vi "Update FormulaG Project.vi"() -> ()   [LabVIEW 2020]
uses:
  dev/Version.ctl
  dev/Updater State.ctl
  c5f3ca88-f85c-4b21-a54c-2e2b82621a56.vi
  fab92dee-f5cc-474f-8dc6-a01214f8643b.vi
  <vilib>/Comparison/Equal/Equal Functor/Equal Functor.lvclass
panel:
  out "Web Folder":path
  out "Project":refnum<vi>
  out "Template Vers Str":string
  out "Project Vers Str":string
  out "Template Version":T1
  out "Project Version":T1
  out "Common Folder":path
  out "Progress":u16(slide) scale=0.0..100.0
  out "Status":string
  out "Players":path[](array[path])
  out "Template":path
  out "Engine Folder":path
  out "Project Path":path
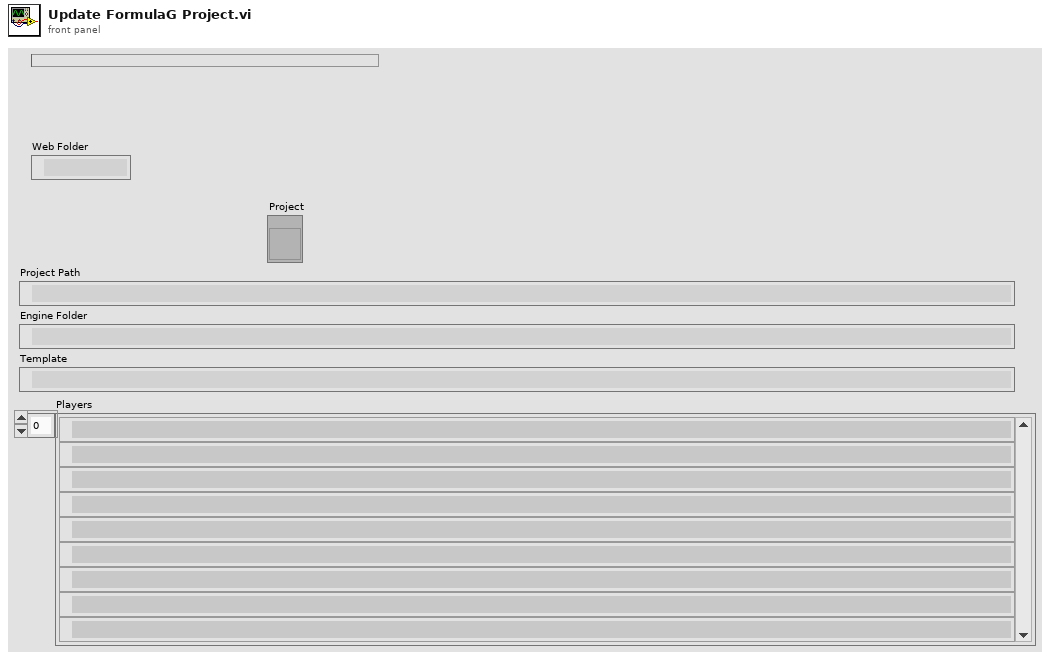
[diagram p1: front panel]
types:
  T1 = typedef "Version.ctl" = cluster{"Major":u16, "Minor":u16, "Fix":u16, "Build":u16}
  T2 = typedef "Updater State.ctl" = enum16{"Get References", "Check Versions", "Confirm", "Close Project", "Copy Engine", "Copy Players", "Open Project", "Version Scripting", "Close"}
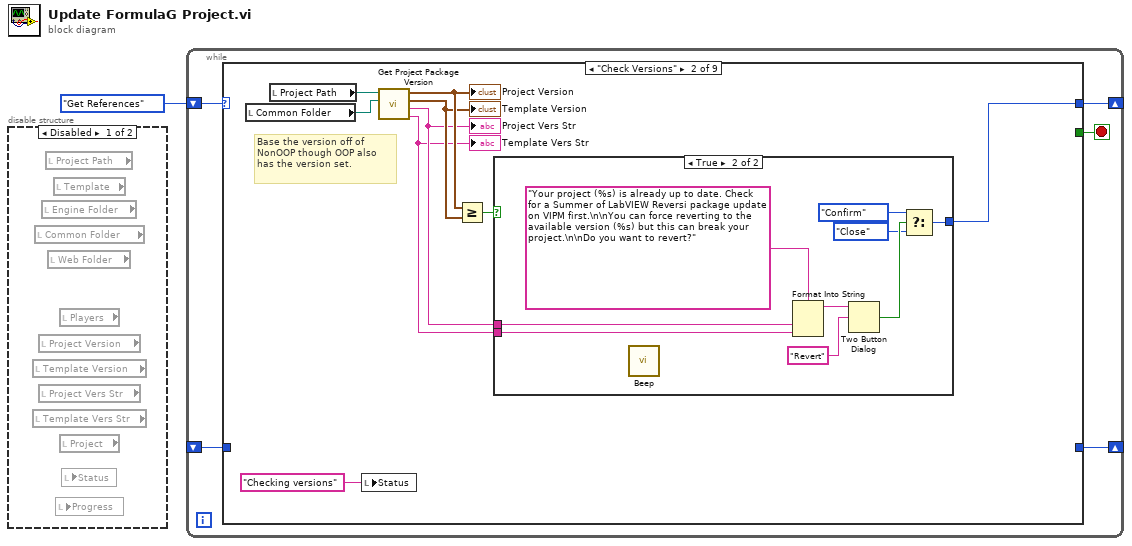
[diagram p0: block diagram]
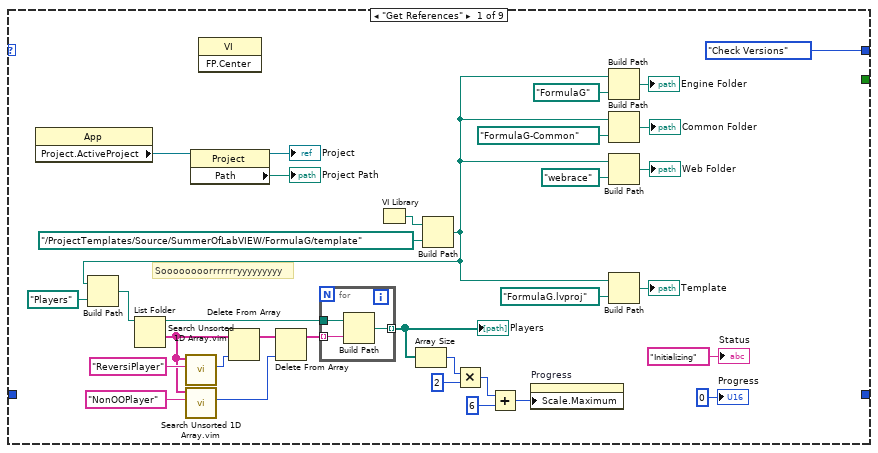
[diagram p3: hidden frame]
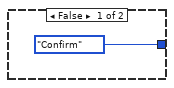
[diagram p4: hidden frame]
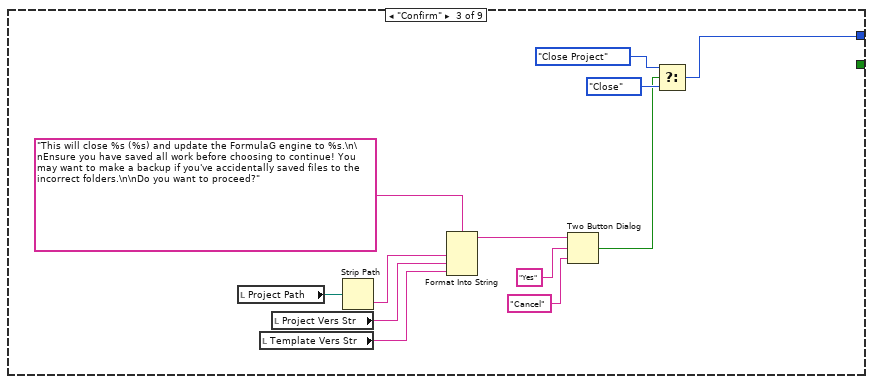
[diagram p5: hidden frame]
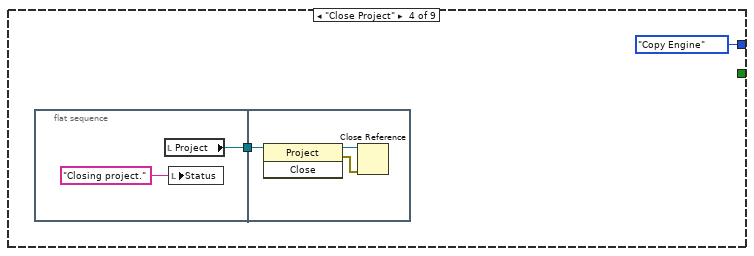
[diagram p6: hidden frame]
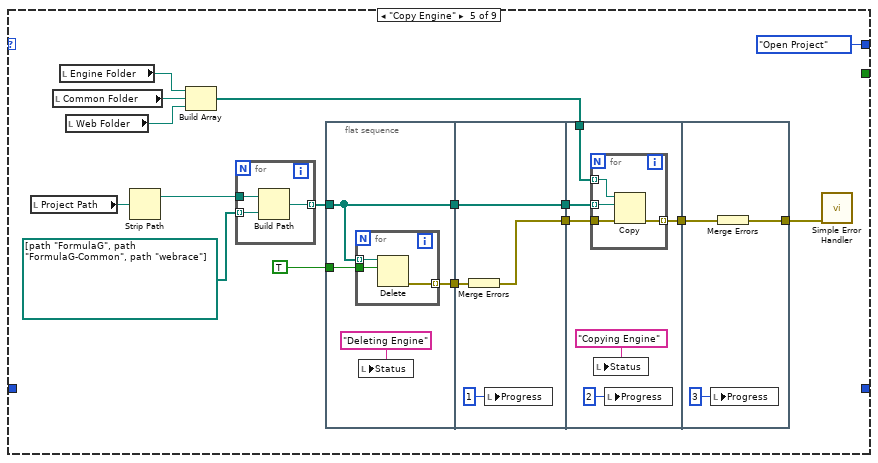
[diagram p7: hidden frame]
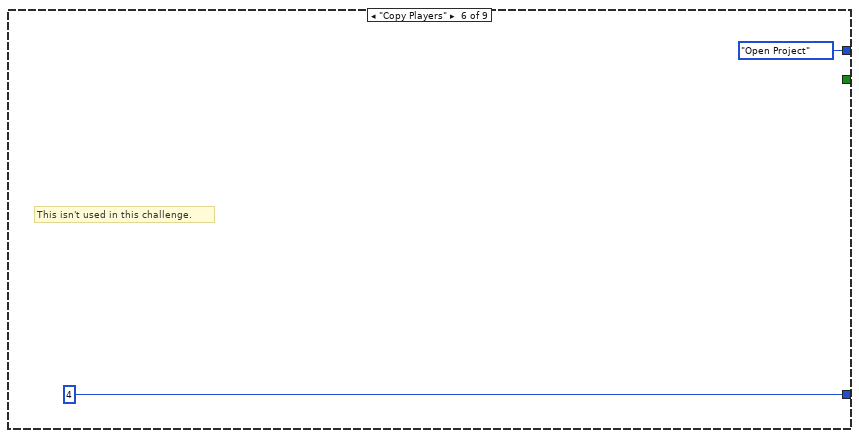
[diagram p8: hidden frame]
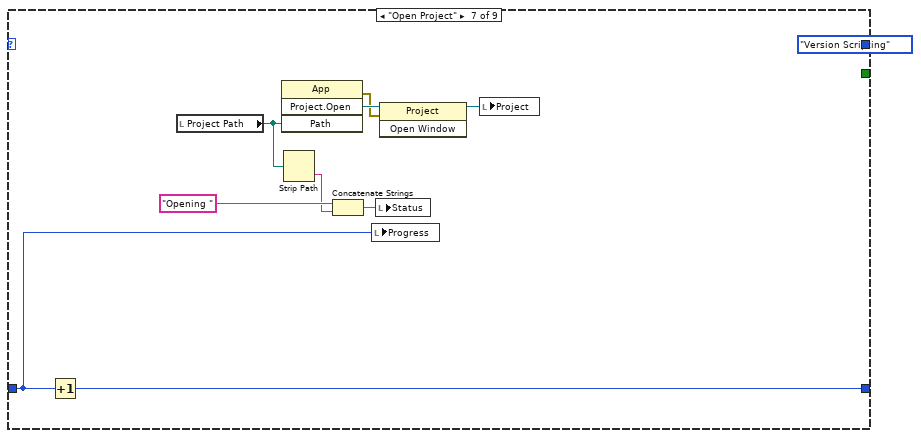
[diagram p9: hidden frame]
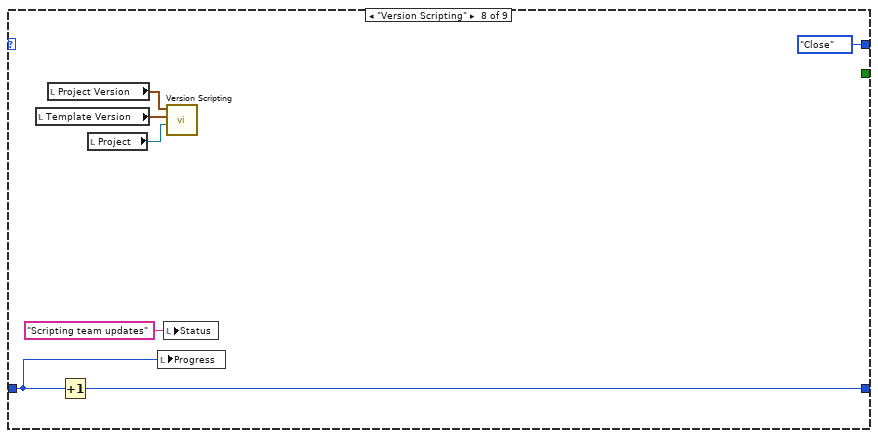
[diagram p10: hidden frame]
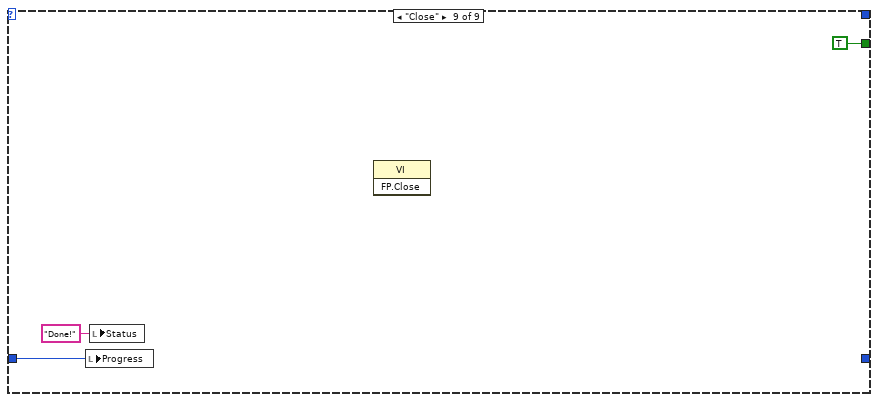
[diagram p11: hidden frame]
diagram:
  n1 = disable-structure shown="Disabled" {
    frame Disabled {
      n2 = local read "Template Version"() -> ()  [unwired: 1 out]
      n3 = local read "Template Vers Str"() -> ()  [unwired: 1 out]
      n4 = local read "Common Folder"() -> ()  [unwired: 1 out]
      n5 = local read "Project Version"() -> ()  [unwired: 1 out]
      n6 = local read "Project Vers Str"() -> ()  [unwired: 1 out]
      n7 = local read "Engine Folder"() -> ()  [unwired: 1 out]
      n8 = local read "Project Path"() -> ()  [unwired: 1 out]
      n9 = local read "Web Folder"() -> ()  [unwired: 1 out]
      n10 = local read "Template"() -> ()  [unwired: 1 out]
      n11 = local read "Progress"() -> ()  [unwired: 1 in]
      n12 = local read "Players"() -> ()  [unwired: 1 out]
      n13 = local read "Project"() -> ()  [unwired: 1 out]
      n14 = local read "Status"() -> ()  [unwired: 1 in]
    }
    frame Enabled {
    }
  }
  n15 = while {
    shift-right: [w5] -> _
    shift-left: Updater_State."Get References" -> [w6]
    shift-right: [w3] -> _
    shift-left: _ -> [w2]
    stop <- w4 stop-if-true
    n16 = case shown="\"Check Versions\"" w6 {
      tunnel: [Updater_State."Check Versions" ("f") w45 w68 Updater_State."Copy Engine" ("f") Updater_State."Open Project" ("f") Updater_State."Open Project" ("f") Updater_State."Version Scripting" ("f") Updater_State."Close" ("f") _] -> w5
      tunnel: [_ _ _ _ _ _ _ _ TRUE] -> w4
      tunnel: [_ _ _ _ _ u16 4 ("Progress") w127 w136 _] -> w3
      tunnel: w2 -> [_ _ _ _ _ _ w128 w137 w144]
      frame "Get References" {
        # "Soooooooorrrrrrryyyyyyyyy"
        n17 = property class="App"() -> ("Project.ActiveProject"=w17:refnum<vi>)  [unwired: 2 in, 2 out]
        n18 = property class="Project"(reference=w17) -> (reference out=→"Project":refnum<vi>, "Path"=→"Project Path":path)  [unwired: 1 in, 1 out]
        n19 = invoke class="VI" method="FP.Center"() -> ()  [unwired: 3 in, 3 out]
        n20 = VI Library() -> (path=w37:path)
        n21 = Build Path(base path=w37, name or relative path=path "../ProjectTemplates/Source/SummerOfLabVIEW/FormulaG/template") -> (appended path=w7:path)
        n22 = Build Path(base path=w7, name or relative path=path "Players") -> (appended path=w30:path)
        n23 = List Folder(path=w30) -> (path out=w27:path, folder names=w13:string[])  [unwired: 3 in, 2 out]
        n24 = call "Search Unsorted 1D Array.vim"("element"="ReversiPlayer", "unsorted 1D array"=w13) -> ("index of element"=w28:i32)  [unwired: 9 in]
        n25 = call "Search Unsorted 1D Array.vim"("element"="NonOOPlayer", "unsorted 1D array"=w13) -> ("index of element"=w11:i32)  [unwired: 9 in]
        n26 = Delete From Array(array=w13, index=w28) -> (array with subset deleted=w12:string[])  [unwired: 1 in, 1 out]
        n27 = Delete From Array(array=w12, index=w11) -> (array with subset deleted=w10:string[])  [unwired: 1 in, 1 out]
        n28 = for {
          tunnel: w10 -> [w41] mode=indexing
          tunnel: w27 -> [w42]
          tunnel: [w40] -> w25 mode=indexing
          n29 = Build Path(base path=w42, name or relative path=w41) -> (appended path=w40:path)
        }
        "Players" <- w25
        n30 = Array Size(array=w25) -> (size(s)=w24:i32)
        n31 = Multiply(x=w24, y=2) -> (x*y=w22:i32)
        n32 = Add(x=w22, y=6) -> (x+y=w20:i32)
        n33 = property on="Progress" class="Slide (strict)"("Scale.Maximum"=w20) -> ()  [unwired: 2 in, 2 out]
        n34 = Build Path(base path=w7, name or relative path=path "FormulaG") -> (appended path=→"Engine Folder":path)
        n35 = Build Path(base path=w7, name or relative path=path "FormulaG-Common") -> (appended path=→"Common Folder":path)
        n36 = Build Path(base path=w7, name or relative path=path "webrace") -> (appended path=→"Web Folder":path)
        n37 = Build Path(base path=w7, name or relative path=path "FormulaG.lvproj") -> (appended path=→"Template":path)
        "Status" <- "Initializing" ("Status")
        "Progress" <- u16 0 ("Progress")
      }
      frame "Check Versions" {
        # "Base the version off of NonOOP though OOP also has the version set."
        n38 = local read "Common Folder"() -> (w49:path)
        n39 = local read "Project Path"() -> (w51:path)
        n40 = local write "Status"("Checking versions" ("Status")) -> ()
        n41 = call "Get Project Package Version.vi"("Template Project"=w49, "Project Path"=w51) -> ("Template Vers Str"=w43:string, "Project Vers Str"=w44:string, "Template Version"=w47:T1, "Project Version"=w48:T1)  [unwired: 6 in]
        "Project Version" <- w48
        "Template Version" <- w47
        "Project Vers Str" <- w44
        "Template Vers Str" <- w43
        n42 = Greater Or Equal?(x=w48, y=w47) -> (x >= y?=w46:bool)
        n43 = case shown="True" w46 {
          tunnel: [Updater_State."Confirm" ("f") w53] -> w45
          tunnel: w44 -> [_ w60]
          tunnel: w43 -> [_ w59]
          frame False {
          }
          frame True {
            n44 = call <vilib>:"Beep.vi"() -> ()  [unwired: 12 in]
            n45 = Format Into String(format string="Your project (%s) is already up to date. Check for a Summer of LabVIEW Reversi package update on VIPM first.\n\nYou can force reverting to the available version (%s) but this can break your project.\n\nDo you want to revert?" ("message"), w60, w59) -> (resulting string=w58:string)  [unwired: 2 in, 1 out]
            n46 = Two Button Dialog(message=w58, 2:"Revert" ("T button name (\"OK\")")) -> (T button?=w56:bool)  [unwired: 1 in]
            n47 = Select(t=Updater_State."Confirm" ("f"), s=w56, f=Updater_State."Close") -> (s? t:f=w53:T2)
          }
        }
      }
      frame "Confirm" {
        n48 = local read "Project Path"() -> (w66:path)
        n49 = local read "Template Vers Str"() -> (w62:string)
        n50 = local read "Project Vers Str"() -> (w63:string)
        n51 = Strip Path(path=w66) -> (name=w65:string)  [unwired: 1 out]
        n52 = Format Into String(format string="This will close %s (%s) and update the FormulaG engine to %s.\n\nEnsure you have saved all work before choosing to continue! You may want to make a backup if you've accidentally saved files to the incorrect folders.\n\nDo you want to proceed?" ("message"), w65, w63, w62) -> (resulting string=w64:string)  [unwired: 2 in, 1 out]
        n53 = Two Button Dialog(message=w64, 1:"Cancel" ("F button name (\"Cancel\")"), 2:"Yes" ("T button name (\"OK\")")) -> (T button?=w69:bool)
        n54 = Select(t=Updater_State."Close Project", s=w69, f=Updater_State."Close") -> (s? t:f=w68:T2)
      }
      frame "Close Project" {
        n55 = flat-sequence {
          tunnel: [w76] -> w74
          tunnel: w74 -> [w78]
          frame #0 {
            n56 = local read "Project"() -> (w76:refnum<vi>)
            n57 = local write "Status"("Closing project." ("Status")) -> ()
          }
          frame #1 {
            n58 = invoke class="Project" method="Close"(reference=w78) -> (reference out=w80:refnum<vi>, error out=w79:errorcluster)  [unwired: 2 in, 1 out]
            n59 = Close Reference(reference=w80, error in (no error)=w79) -> ()  [unwired: 1 out]
          }
        }
      }
      frame "Copy Engine" {
        n60 = local read "Project Path"() -> (w96:path)
        n61 = local read "Common Folder"() -> (w86:path)
        n62 = local read "Engine Folder"() -> (w85:path)
        n63 = local read "Web Folder"() -> (w84:path)
        n64 = Strip Path(path=w96) -> (stripped path=w95:path)  [unwired: 1 out]
        n65 = Build Array(w85, w86, w84) -> (w81:path[])
        n66 = for {
          tunnel: path[] [path "FormulaG", path "FormulaG-Common", path "webrace"] -> [w97] mode=indexing
          tunnel: w95 -> [w99]
          tunnel: [w98] -> w94 mode=indexing
          n67 = Build Path(base path=w99, name or relative path=w97) -> (appended path=w98:path)
        }
        n68 = flat-sequence {
          tunnel: w94 -> [w100]
          tunnel: [w103] -> w92
          tunnel: [w100] -> w91
          tunnel: TRUE ("entire hierarchy (F)") -> [w101]
          tunnel: w92 -> [w108]
          tunnel: w91 -> [w110]
          tunnel: [w110] -> w90
          tunnel: [w107] -> w89
          tunnel: w90 -> [w115]
          tunnel: w89 -> [w116]
          tunnel: [w114] -> w88
          tunnel: w81 -> [w111]
          tunnel: w88 -> [w122]
          tunnel: [w121] -> w87
          frame #0 {
            n69 = for {
              tunnel: [w106] -> w103 mode=indexing
              tunnel: w101 -> [w105]
              tunnel: w100 -> [w104] mode=indexing
              n70 = Delete(path (use dialog)=w104, entire hierarchy (F)=w105) -> (error out=w106:errorcluster)  [unwired: 3 in, 2 out]
            }
            n71 = local write "Status"("Deleting Engine") -> ()
          }
          frame #1 {
            n72 = Merge Errors(w108) -> (w107:errorcluster)
            n73 = local write "Progress"(u16 1 ("Progress")) -> ()
          }
          frame #2 {
            n74 = for {
              tunnel: w115 -> [w119] mode=indexing
              tunnel: w116 -> [w120]
              tunnel: [w118] -> w114 mode=indexing
              tunnel: w111 -> [w117] mode=indexing
              n75 = Copy(8:w120, 10:w119, 11:w117) -> (0:w118:errorcluster)  [unwired: 2 in, 2 out]
            }
            n76 = local write "Status"("Copying Engine") -> ()
            n77 = local write "Progress"(u16 2 ("Progress")) -> ()
          }
          frame #3 {
            n78 = local write "Progress"(u16 3 ("Progress")) -> ()
            n79 = Merge Errors(w122) -> (w121:errorcluster)
          }
        }
        n80 = call <vilib>:"Simple Error Handler.vi"("error in (no error)"=w87) -> ()  [unwired: 4 in, 5 out]
      }
      frame "Copy Players" {
        # "This isn't used in this challenge."
      }
      frame "Open Project" {
        n81 = Increment(x=w128) -> (x+1=w127:u16)
        n82 = local read "Project Path"() -> (w132:path)
        n83 = invoke class="App" method="Project.Open"("Path"=w132) -> (error out=w133:errorcluster, "Project:Open"=w134:refnum<vi>)  [unwired: 3 in, 2 out]
        n84 = Strip Path(path=w132) -> (name=w130:string)  [unwired: 1 out]
        n85 = Concatenate Strings("Opening " ("Status"), w130) -> (w129:string)
        n86 = local write "Progress"(w128) -> ()
        n87 = local write "Status"(w129) -> ()
        n88 = invoke class="Project" method="Open Window"(reference=w134, error in=w133) -> (reference out=w126:refnum<vi>)  [unwired: 1 in, 2 out]
        n89 = local write "Project"(w126) -> ()
      }
      frame "Version Scripting" {
        n90 = local read "Template Version"() -> (w142:T1)
        n91 = local read "Project Version"() -> (w141:T1)
        n92 = Increment(x=w137) -> (x+1=w136:u16)
        n93 = local read "Project"() -> (w140:refnum<vi>)
        n94 = local write "Progress"(w137) -> ()
        n95 = local write "Status"("Scripting team updates" ("Status")) -> ()
        n96 = call "Version Scripting.vi"("Project"=w140, "To"=w142, "From"=w141) -> ()  [unwired: 9 in]
      }
      frame "Close" {
        n97 = local write "Progress"(w144) -> ()
        n98 = local write "Status"("Done!" ("Status")) -> ()
        n99 = invoke class="VI" method="FP.Close"() -> ()  [unwired: 3 in, 3 out]
      }
    }
  }
